vi "DIGIT_5122_Write_Data.vi"(7 "Accum Number":i16, 8 "error in (no error)":errorcluster, 9 "dataset":i16[][](array[numeric]), 10 "wfm info":T2, 11 "SOFTWARE Inputs":T3={"Application Directory"=path "D:/S.O.F.T.S/LABVIEW/PIL", "Resources Path"=path "D:/S.O.F.T.S/LABVIEW/PIL/resources", "Data Path"=path "D:/PIRENEA/DATA", "XML Path"=path "D:/PIRENEA/DATA", "XML File Filter"="*.xml", "Excit Scripts Path"=path "D:/PIRENEA/EXCIT_SCRIPTS", "Excit Scripts File Filter"="*.txt", "Excit Waveforms Path"=path "D:/PIRENEA/EXCIT_WFMS", "Excit Waveforms File Filter"="*.bin", "Timing Scripts Path"=path "D:/PIRENEA/TIMING_SCRIPTS", "Timing Scripts File Filter"="*.txt", "Timing Waveforms Path"=path "D:/PIRENEA/TIMING_WFMS", "Timing Waveforms File Filter"="*.bin", "Trapping Waveforms Path"=path "D:/PIRENEA/TRAPPING_WFMS", "Trapping Waveforms File Filter"="*.bin"}) -> (0 "error out":errorcluster, 2 "Frequency Spectrum":T1(array[cluster]), 3 "Dataset Signal":cluster{sgl[], sgl[]}[](array[cluster]))   [LabVIEW 2015]
doc: "This VI writes a raw dataset into a disk file with the format :\n- number of points (one I16)\n- data (I16 points)\n- 1/sample rate, i.e. time step (one DBL)\n- vertical range (one DBL)\n\nThe file naming convention is :\nyyyy_mm_dd_xxx.A00 for the first acqusisition,\nyyyy_mm_dd_xxx.B00 for the second, etc."
uses:
  controls/SOFTWARE_Inputs.ctl
panel:
  out "nouveau chemin":path
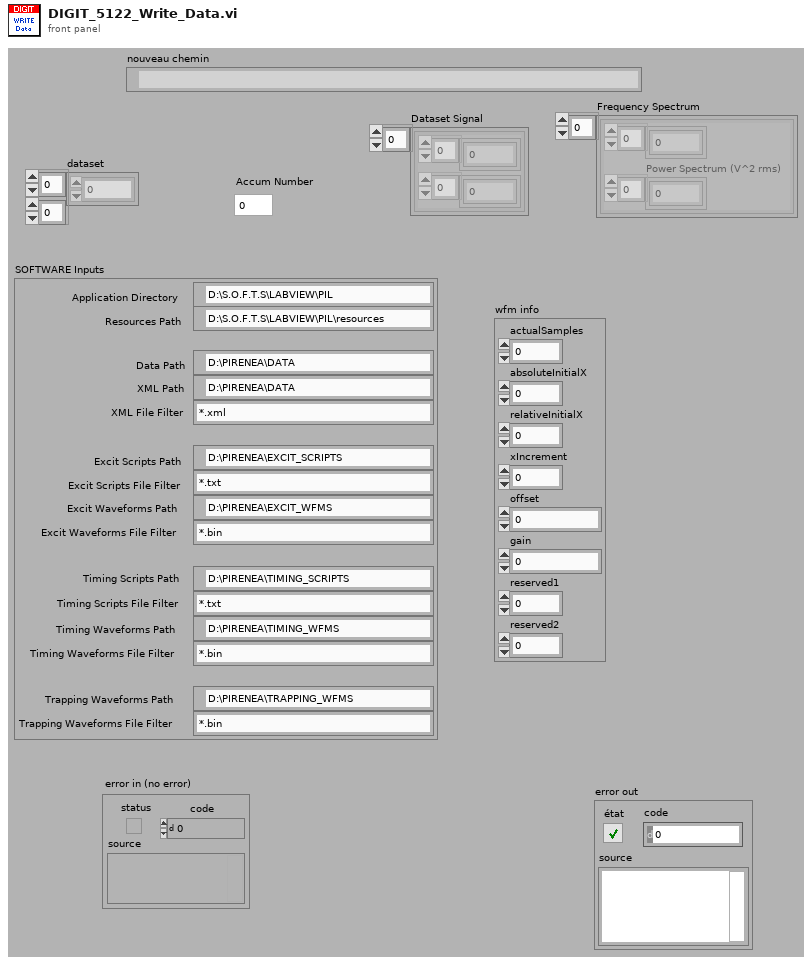
[diagram p1: front panel]
types:
  T1 = cluster{dbl[], "Power Spectrum (V^2 rms)":dbl[]}[]
  T2 = cluster{"actualSamples":i32, "absoluteInitialX":dbl, "relativeInitialX":dbl, "xIncrement":dbl, "offset":dbl, "gain":dbl, "reserved1":dbl, "reserved2":dbl}
  T3 = typedef "SOFTWARE_Inputs.ctl" = cluster{"Application Directory":path, "Resources Path":path, "Data Path":path, "XML Path":path, "XML File Filter":string, "Excit Scripts Path":path, "Excit Scripts File Filter":string, "Excit Waveforms Path":path, "Excit Waveforms File Filter":string, "Timing Scripts Path":path, "Timing Scripts File Filter":string, "Timing Waveforms Path":path, "Timing Waveforms File Filter":string, "Trapping Waveforms Path":path, "Trapping Waveforms File Filter":string}
  T4 = enum16{"big-endian, network order", "native, host order", "little-endian"}
  T5 = enum16{"open", "replace", "create", "open or create", "replace or create", "replace or create with confirmation"}
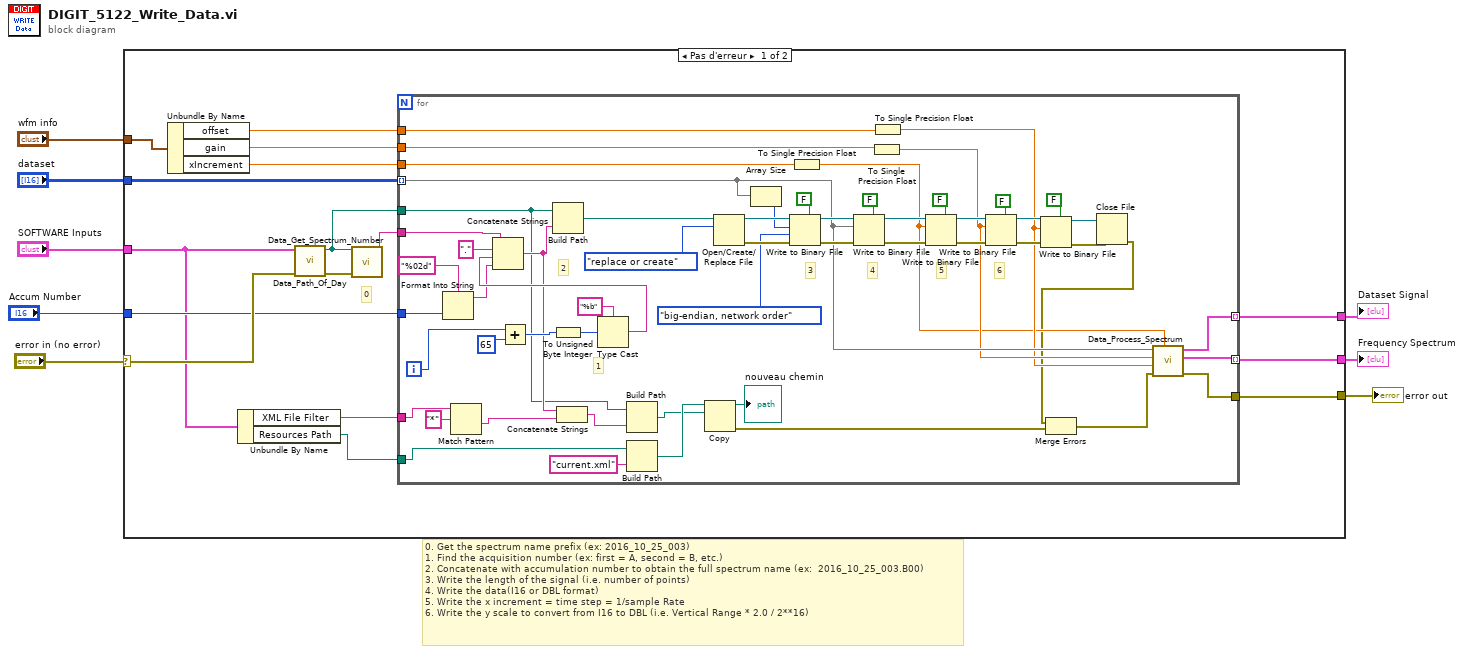
[diagram p0: block diagram]
diagram:
  # "0. Get the spectrum name prefix (ex: 2016_10_25_003)\n1. Find the acquisition number (ex: first = A, second = B, etc.)\n2. Concatenate with accumulation number to obtain the full spectrum name (ex:  2016_10_25_003.B00)\n3. Write the length of the signal (i.e. number of points)\n4. Write the data(I16 or DBL format)\n5. Write the x increment = time step = 1/sample Rate\n6. Write the y scale to convert from I16 to DBL (i.e. Vertical Range * 2.0 / 2**16)"
  n1 = case shown="Pas d'erreur" "error in (no error)" {
    selector: "error in (no error)" -> [w21 w81]
    tunnel: [w14 w81] -> w3
    tunnel: "SOFTWARE Inputs" -> [w11 _]
    tunnel: "Accum Number" -> [w20 _]
    tunnel: "dataset" -> [w19 _]
    tunnel: "wfm info" -> [w18 _]
    tunnel: [w13 _] -> w2
    tunnel: [w12 _] -> w1
    frame No Error {
      # "0"
      n2 = Unbundle By Name(w18) -> ("offset"=w17:dbl, "gain"=w16:dbl, "xIncrement"=w15:dbl)
      n3 = Unbundle By Name(w11) -> ("XML File Filter"=w10:string, "Resources Path"=w9:path)
      n4 = call "Data_Path_Of_Day.vi"("error in (no error)"=w21, "SOFTWARE Inputs"=w11) -> ("error out"=w24:errorcluster, "Path of the Day"=w22:path)  [unwired: 8 in]
      n5 = call "Data_Get_Spectrum_Number.vi"("error in (no error)"=w24, "Path of the Day"=w22) -> ("Next Spectrum Number"=w23:string)  [unwired: 7 in, 2 out]
      n6 = for {
        tunnel: w23 -> [w76]
        tunnel: w22 -> [w34]
        tunnel: w20 -> [w59]
        tunnel: w19 -> [w46] mode=indexing
        tunnel: w17 -> [w48]
        tunnel: w16 -> [w50]
        tunnel: w15 -> [w51]
        tunnel: [w43] -> w13 mode=indexing
        tunnel: [w42] -> w14
        tunnel: [w41] -> w12 mode=indexing
        tunnel: w10 -> [w37]
        tunnel: w9 -> [w32]
        i -> [w70]
        # "6"
        # "5"
        # "4"
        # "3"
        # "2"
        # "1"
        n7 = Format Into String(format string="%02d" ("chaîne de format"), w59) -> (resulting string=w68:string)  [unwired: 2 in, 1 out]
        n8 = Match Pattern(string=w37, regular expression="*" ("expression régulière")) -> (after substring=w35:string)  [unwired: 1 in, 3 out]
        n9 = Add(x=w70, y=i16 65) -> (x+y=w77:i32)
        n10 = To Unsigned Byte Integer(number=w77) -> (unsigned 8bit integer=w78:u8)
        n11 = Type Cast(type="%b", x=w78) -> (*(type *) &x=w74:string)
        n12 = Concatenate Strings(w76, "." ("chaîne"), w74, w68) -> (w38:string)
        n13 = Build Path(base path=w34, name or relative path=w38) -> (appended path=w71:path)
        n14 = Concatenate Strings(w38, w35) -> (w33:string)
        n15 = Build Path(base path=w34, name or relative path=w33) -> (appended path=w26:path)
        n16 = Build Path(base path=w32, name or relative path="current.xml" ("nom ou chemin relatif")) -> (appended path=w27:path)
        n17 = Copy(10:w26, 11:w27) -> (0:w30:errorcluster, 3:→"nouveau chemin":path)  [unwired: 3 in, 1 out]
        n18 = Open/Create/Replace File(file path (use dialog)=w71, operation (0:open)=T5."replace or create" ("opération (0 : open)")) -> (refnum out=w67:refnum<file>, error out=w66:errorcluster)  [unwired: 4 in, 1 out]
        n19 = Array Size(array=w46) -> (size(s)=w47:i32)
        n20 = Write to Binary File(file (use dialog)=w67, data=w47, error in=w66, 5:FALSE ("ajouter une taille de tableau ou de chaîne ? (V)"), 9:T4."big-endian, network order" ("ordre des octets (0 : big-Endian, network order)")) -> (refnum out=w63:refnum<file>, error out=w64:errorcluster)  [unwired: 1 in, 1 out]
        n21 = To Single Precision Float(number=w51) -> (single precision float=w39:sgl)
        n22 = Write to Binary File(file (use dialog)=w63, data=w46, error in=w64, 5:FALSE ("ajouter une taille de tableau ou de chaîne ? (V)")) -> (refnum out=w61:refnum<file>, error out=w62:errorcluster)  [unwired: 2 in, 1 out]
        n23 = To Single Precision Float(number=w50) -> (single precision float=w45:sgl)
        n24 = To Single Precision Float(number=w48) -> (single precision float=w44:sgl)
        n25 = Write to Binary File(file (use dialog)=w61, data=w39, error in=w62, 5:FALSE ("ajouter une taille de tableau ou de chaîne ? (V)")) -> (refnum out=w57:refnum<file>, error out=w58:errorcluster)  [unwired: 2 in, 1 out]
        n26 = Write to Binary File(file (use dialog)=w57, data=w45, error in=w58, 5:FALSE ("ajouter une taille de tableau ou de chaîne ? (V)")) -> (refnum out=w54:refnum<file>, error out=w55:errorcluster)  [unwired: 2 in, 1 out]
        n27 = Write to Binary File(file (use dialog)=w54, data=w44, error in=w55, 5:FALSE ("ajouter une taille de tableau ou de chaîne ? (V)")) -> (refnum out=w53:refnum<file>, error out=w52:errorcluster)  [unwired: 2 in, 1 out]
        n28 = Close File(refnum=w53, error in=w52) -> (error out=w29:errorcluster)  [unwired: 1 out]
        n29 = Merge Errors(w29, w30) -> (w28:errorcluster)
        n30 = call "Data_Process_Spectrum.vi"("wfm info"=w39, "error in"=w28, 9:w44, 10:w45, "dataset"=w46) -> ("error out"=w42:errorcluster, "Frequency Spectrum"=w41:cluster{dbl[], "Power Spectrum (V^2 rms)":dbl[]}, "Dataset Signal"=w43:cluster{sgl[], sgl[]})  [unwired: 4 in]
      }
    }
    frame Error {
    }
  }
  "error out" <- w3
  "Dataset Signal" <- w2
  "Frequency Spectrum" <- w1
